vi "Clear.vi"(8 "error in (no error)":errorcluster, 11 "Ramp Use Case in":refnum<class "Ramp Voltage.lvclass">) -> (0 "error out":errorcluster, 3 "Ramp Use Case out":refnum<class "Ramp Voltage.lvclass">)   [LabVIEW 2020, in "High Level PSU With Tests.lvlib" / "Ramp Voltage.lvclass"]
uses:
  Ramp Voltage.lvclass
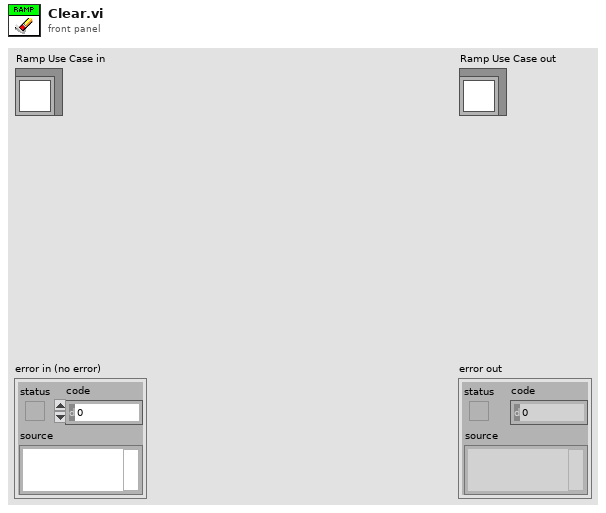
[diagram p1: front panel]
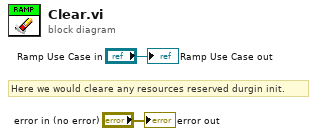
[diagram p0: block diagram]
diagram:
  # "Here we would cleare any resources reserved durgin init."
  "error out" <- "error in (no error)"
  "Ramp Use Case out" <- "Ramp Use Case in"
